vi "SLL DE Reorder Virtual Channels Values_Numeric Array.vi"(8 "error in (no error)":errorcluster, 9 "# Samples":i32, 10 "Channel Order":i32[](array[numeric]), 11 "Disordered DI Data":dbl[][](array[numeric])) -> (0 "error out":errorcluster, 3 "Ordered DI Data":dbl[][](array[numeric]))   [LabVIEW 2013]
doc: "Copyright © 2005, Soliton Technologies.\nAll rights reserved."
uses:
  Controls/SLL DE Virtual Chart Datalog Driver Options.ctl
panel:
  out "logical AND":bool
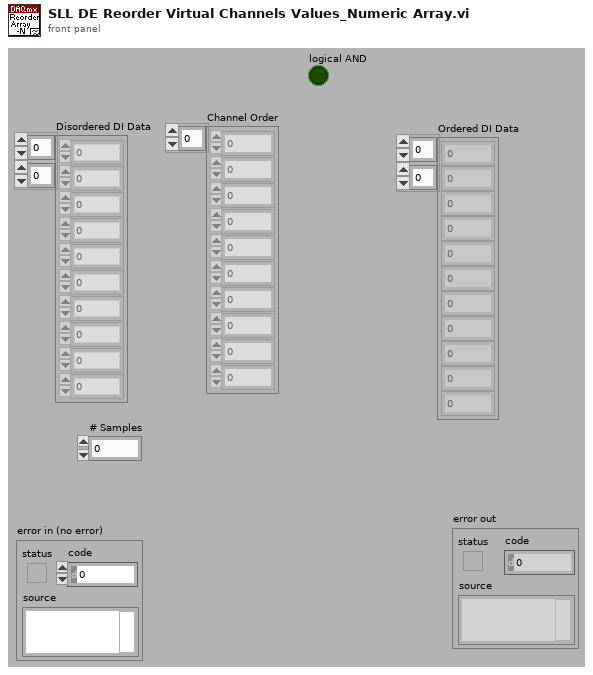
[diagram p1: front panel]
types:
  T1 = typedef "SLL DE Virtual Chart Datalog Driver Options.ctl" = enum16{"Initialise", "Write Headings", "Write", "Check File Size", "Read", "Clear"}
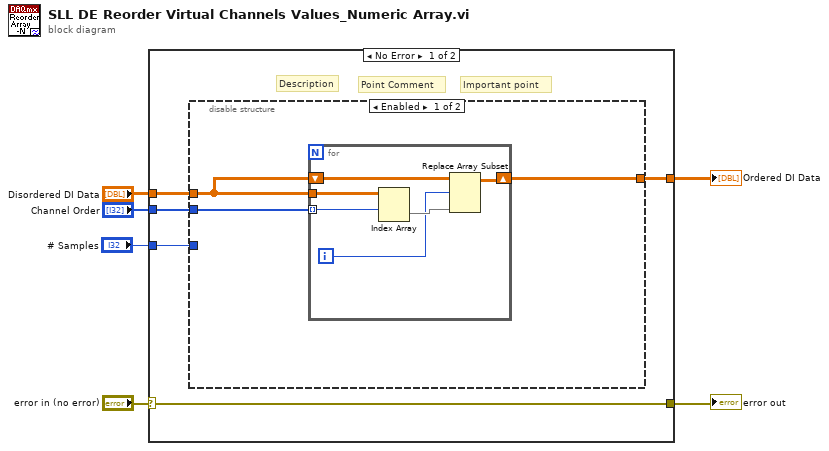
[diagram p0: block diagram]
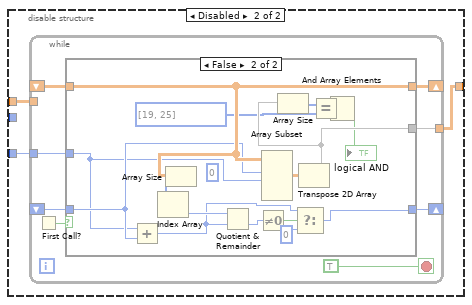
[diagram p2: hidden frame]
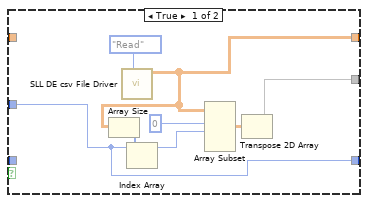
[diagram p3: hidden frame]
diagram:
  n1 = case shown="No Error" "error in (no error)" {
    selector: "error in (no error)" -> [w11 w56]
    tunnel: [w11 w56] -> w5
    tunnel: "Disordered DI Data" -> [w10 w55]
    tunnel: "Channel Order" -> [w9 _]
    tunnel: [w8 w55] -> w2
    tunnel: "# Samples" -> [w7 _]
    frame No Error {
      # "Point Comment"
      # "Important point"
      # "Description"
      n2 = disable-structure shown="Enabled" {
        disable-tunnel: w10 -> [w14 w23]
        disable-tunnel: w9 -> [w13 _]
        disable-tunnel: [w12 w21] -> w8
        disable-tunnel: w7 -> [_ w22]
        frame Enabled {
          n3 = for {
            shift-right: [w15] -> w12
            shift-left: w14 -> [w18]
            tunnel: w14 -> [w20]
            tunnel: w13 -> [w19] mode=indexing
            i -> [w16]
            n4 = Index Array(array=w20, index (row)=w19) -> (element=w17:dbl[])  [unwired: 1 in]
            n5 = Replace Array Subset(array=w18, new element=w17, index (row)=w16) -> (w15:dbl[][])  [unwired: 1 in]
          }
        }
        frame Disabled {
          n6 = while {
            tunnel: w23 -> [_]
            shift-right: [w29] -> _
            shift-left: _ -> [w28]
            tunnel: w22 -> [w27]
            shift-right: [w26] -> _
            shift-left: _ -> [w24]
            tunnel: [w25] -> w21
            stop <- TRUE stop-if-true
            n7 = First Call?() -> (First Call?: T/F=w30:bool)
            n8 = case shown="False" w30 {
              tunnel: [w35 w51] -> w29
              tunnel: w28 -> [_ w51]
              tunnel: w27 -> [w33 w45]
              tunnel: [w33 w46] -> w26
              tunnel: [w32 w43] -> w25
              tunnel: w24 -> [_ w48]
              frame True {
                n9 = call "SLL DE csv File Driver.vi"("Datalog Driver Cases"=SLL_DE_Virtual_Chart_Datalog_Driver_Options."Read") -> ("Data Out"=w35:dbl[][])  [unwired: 6 in, 4 out]
                n10 = Array Size(array=w35) -> (size(s)=w36:i32[])
                n11 = Index Array(array=w36) -> ()  [unwired: 1 in, 1 out]
                n12 = Array Subset(array=w35, index (row)=0 ("index"), length (row)=w33) -> (w34:dbl[][])  [unwired: 2 in]
                n13 = Transpose 2D Array(2D array=w34) -> (transposed array=w32:dbl[][])
              }
              frame False {
                (unwired) 0 ("index")
                n14 = Add(x=w45, y=w48) -> (x+y=w44:i32)
                n15 = Array Size(array=w51) -> (size(s)=w54:i32[])
                n16 = Index Array(array=w54) -> (element=w53:i32)  [unwired: 1 in]
                n17 = Quotient & Remainder(x=w53, y=w44) -> (floor(x/y)=w50:i32)  [unwired: 1 out]
                n18 = Not Equal To 0?(x=w50) -> (x != 0?=w49:bool)
                n19 = Array Subset(array=w51, index (row)=w48, length (row)=w45) -> (w52:dbl[][])  [unwired: 2 in]
                n20 = Select(t=w44, s=w49, f=0) -> (s? t:f=w46:i32)
                n21 = Transpose 2D Array(2D array=w52) -> (transposed array=w43:dbl[][])
                n22 = Array Size(array=w43) -> (size(s)=w42:i32[])
                n23 = Equal?(x=w42, y=i32[] [19, 25]) -> (x = y?=w40:bool[])
                n24 = And Array Elements(Boolean array=w40) -> (logical AND=→"logical AND":bool)
              }
            }
          }
        }
      }
    }
    frame Error {
    }
  }
  "error out" <- w5
  "Ordered DI Data" <- w2
